vi "Set Image.vi"(8 "error in (no error)":errorcluster, 11 "CCDCamera in":refnum<class "iKon-L.lvclass">) -> (0 "error out":errorcluster, 3 "CCDCamera out":refnum<class "iKon-L.lvclass">)   [LabVIEW 2018, in "iKon-L.lvclass"]
doc: "Set the dimensions of the image\n\nWith this function, it is possible to set the inital column, inital line, final column and final line. Also, the vertical and horizontal binning of the pixels can be set."
uses:
  iKon-L.lvclass
  C:/Users/Denis/Desktop/S4ACS/S4ACS/Sim_CCD/Sim_CCD.lvclass
  Sim_CCD/Sim_CCD.lvclass
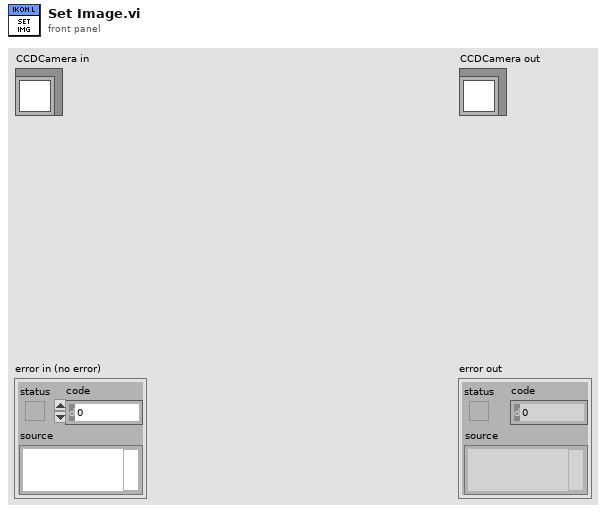
[diagram p1: front panel]
types:
  T1 = cluster{"PREAMP":u16, "READOUT_RATE":u16, "VERTICAL_SHIFT_SPEED":u16, "READ_MODE":u16, "VERTICAL_CLOCK_VOLTAGE":u16, "ACQUISITION_MODE":u16, "AD_CHANNEL":u16, "SHUTTER_TTL":u16, "SHUTTER_OPENING_TIME":u16, "SHUTTER_CLOSING_TIME":u16, "SHUTTER_MODE":u16, "TRIGGER_MODE":u16, "VBIN":u16, "INITIAL_LINE":u16, "INITIAL_COLUMN":u16, "FINAL_LINE":u16, "FINAL_COLUMN":u16, "HBIN":u16}
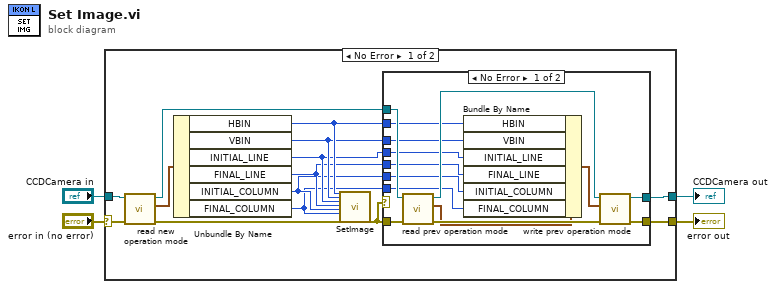
[diagram p0: block diagram]
diagram:
  n1 = case shown="No Error" "error in (no error)" {
    selector: "error in (no error)" -> [w17 w36]
    tunnel: [w13 w36] -> w4
    tunnel: "CCDCamera in" -> [w18 w35]
    tunnel: [w14 w35] -> w3
    frame No Error {
      n2 = call "read new operation mode.vi"("error in (no error)"=w17, "CCDCamera in"=w18) -> ("error out"=w5:errorcluster, "new operation mode"=w16:T1, "CCDCamera out"=w15:refnum<class "iKon-L.lvclass">)  [unwired: 7 in]
      n3 = Unbundle By Name(w16) -> ("HBIN"=w12:u16, "VBIN"=w11:u16, "INITIAL_LINE"=w10:u16, "FINAL_LINE"=w9:u16, "INITIAL_COLUMN"=w8:u16, "FINAL_COLUMN"=w7:u16)
      n4 = call <userlib>:"SetImage.vi"("hbin"=w12, "vbin"=w11, "hstart"=w10, "hend"=w9, "vstart"=w8, "vend"=w7, "error in (no error)"=w5) -> ("error out"=w6:errorcluster)  [unwired: 19 in, 1 out]
      n5 = case shown="No Error" w6 {
        tunnel: w15 -> [w32 w34]
        tunnel: w6 -> [w31 w33]
        tunnel: [w29 w34] -> w14
        tunnel: [w27 w33] -> w13
        tunnel: w12 -> [w24 _]
        tunnel: w11 -> [w23 _]
        tunnel: w10 -> [w22 _]
        tunnel: w9 -> [w21 _]
        tunnel: w8 -> [w20 _]
        tunnel: w7 -> [w19 _]
        frame No Error {
          n6 = call "read prev operation mode.vi"("error in (no error)"=w31, "Simulated_CCD_Camera in"=w32) -> ("error out"=w28:errorcluster, "prev operation mode"=w26:T1, "Simulated_CCD_Camera out"=w30:refnum<class "iKon-L.lvclass">)  [unwired: 7 in]
          n7 = Bundle By Name(cluster=w26, "HBIN"=w24, "VBIN"=w23, "INITIAL_LINE"=w22, "FINAL_LINE"=w21, "INITIAL_COLUMN"=w20, "FINAL_COLUMN"=w19) -> (w25:T1)
          n8 = call "write prev operation mode.vi"("error in (no error)"=w28, "prev operation mode"=w25, "Simulated_CCD_Camera in"=w30) -> ("error out"=w27:errorcluster, "Simulated_CCD_Camera out"=w29:refnum<class "iKon-L.lvclass">)  [unwired: 7 in]
        }
        frame Error {
        }
      }
    }
    frame Error {
    }
  }
  "error out" <- w4
  "CCDCamera out" <- w3
